vi "WS1050 16 DUT VSA-CV Sweep HD_Cycling_Ver1.2.vi"() -> ()   [LabVIEW 2012]
uses:
  WS_VCAP Driver 024/Source/WSVCAP Shell/Type Defs/WSVCAP SHL I2C DUT Mask Mode Enum.ctl
  <vilib>/Utility/file.llb/Read From Spreadsheet File (DBL).vi
panel:
  out "VISA resource name out":refnum<visa-resource-name>="GPIB0::3::INSTR"
  out "date string":string="5/19/2014"
  out "PS1 Out":refnum<visa-resource-name>
  out "Ke2000 Out":refnum<visa-resource-name>="GPIB0::9::INSTR"
  in  "Tab Control":enum32{"Inst Control", "Data Output", "Graphs"}(tab)
  in  "Bank to Stress":u16(ring) items=["All OFF", "All ON", "Bank_C1", "Bank_C2", "Bank_C3"]
  out "AD7747 Values":string[][](table)
  in  "Lot#":string="4NEMB"
  in  "Wafer#":string="20-EB"
  in  "File Name":string="HD_4NEMB_25_EB_65C_44V_100DC_BRD2_150916_1"
  in  "TMN DC\\CAP Data Log File Path":path=path "C:/WS1050 16 DUT Data"
  in  "SN":string[](array[string])=["1", "2", "3", "4", "5", "6", "7", "8", "9", "10", "11", "12", "13", "14", "15", "16"]
  in  "Test Program":string="WS1050 16 DUT VSA_CV Sweep HD_Cycling Ver1.2"
  out "Current Date":string="8/28/2014"
  out "Current Time":string="0950"
  in  "Start Date":string="4/24/2014"
  in  "Start Time":string="1542"
  in  "Comment":string="VSA CV Sweep"
  in  "OK Button":bool
  in  "Calibration":bool
  in  "Control Setting":bool
  in  "CP Setting":i32(ring) items=["CP OFF", "CP ON", "CP 35V", "CP 40V", "CP 44V", "CP 50V", "DVA OFF", "DVA ON", "Reg1 ON", "Reg1 OFF", "Reg2 ON", "Reg2 OFF", "Reg3 ON", "Reg3 OFF"]
  in  "VDD(V)":dbl=3.3 format="%.3g"
  in  "SPI Clock Rate (Hz)":dbl=1000000.0 caption="Meas Speed" format="%.1p Hz"
  out "AR  Measurent(Hz)":dbl
  in  "PS1 Source":refnum<visa-resource-name>="GPIB0::5::INSTR"
  in  "Ke2000":refnum<visa-resource-name>="GPIB0::9::INSTR"
  out "Simulate FPGA":bool
  out "Online":bool
  in  "Ke2400":refnum<visa-resource-name>="GPIB0::3::INSTR"
  in  "Initialize AD7747":bool
  in  "DUT Mask Mode":T1=enum."All"
  in  "RFFE Slave Address":u8=7 caption="Slave Address" format="0x%02x"
  out "Activity Log":string="05/19/2014 -- 12:24:35.853::WSVCAP::APP::Application Started\n05/19/2014 -- 12:24:37.606::WSVCAP::WSVCAP SHL::WR I2C-REG:0x0A;MASK:0xFFFFFFFFFFFF;C1 DATA:22:22:22:22:22:22:22:22:22:22:22:22:22:22:22:22;C2 DATA:22:22:22:22:22:22:22:22:22:22:22:22:22:22:22:22;C3 DATA:22:22:22:22:22:22:22:22:22:22:22:22:22:22:22:22\r\n05/19/2014 -- 12:24:37.773::WSVCAP::WSVCAP SHL::WR I2C-ST:0,0,4,1\r\n05/19/2014 -- 12:24:37.903::WSVCAP::WSVCAP SHL::RD I2C-BYTES:4;ADD:0x00;MASK:0xFFFFFFFFFFFF\r\n05/19/2014 -- 12:24:38.045::WSVCAP::WSVCAP SHL::RD I2C:C1 DATA:2:2:2:2:2:2:2:2:2:2:2:2:2:2:2:2|A7:A9:AA:82:82:7F:82:81:82:81:83:82:81:82:82:81|46:36:BB:88:44:A3:E9:2B:32:20:ED:25:BB:3D:68:B|2C:6A:EB:A7:22:56:FE:CC:36:82:D7:B0:3B:48:F9:CC;C2 DATA:2:2:2:2:2:2:2:2:2:2:2:2:2:2:2:2|94:94:94:80:80:80:80:80:81:7E:7E:81:80:7E:80:80|47:33:15:82:62:B:E8:1C:D7:C3:7D:41:7C:B7:4C:2A|C4:B4:AE:8:1E:D1:4E:37:11:C0:6F:63:42:9D:63:B5;C3 DATA:2:2:2:2:2:2:2:2:2:2:2:2:2:2:2:2|95:95:95:81:81:7E:81:80:84:7D:80:83:81:7E:7F:80|AB:C4:14:B5:7B:52:DF:C9:79:5D:5F:30:99:31:1E:F4|6E:5C:F7:A8:C3:EB:7B:EF:33:92:89:77:4D:67:75:DD;STATUS:0:0:4:0\r\n05/19/2014 -- 12:24:38.046::WSVCAP::WSVCAP SHL::WR I2C-REG:0x0A;MASK:0xFFFFFFFFFFFF;C1 DATA:22:22:22:22:22:22:22:22:22:22:22:22:22:22:22:22;C2 DATA:22:22:22:22:22:22:22:22:22:22:22:22:22:22:22:22;C3 DATA:22:22:22:22:22:22:22:22:22:22:22:22:22:22:22:22\r\n05/19/2014 -- 12:24:38.089::WSVCAP::WSVCAP SHL::WR I2C-ST:0,0,4,1\r\n05/19/2014 -- 12:24:38.219::WSVCAP::WSVCAP SHL::RD I2C-BYTES:4;ADD:0x00;MASK:0xFFFFFFFFFFFF\r\n05/19/2014 -- 12:24:38.362::WSVCAP::WSVCAP SHL::RD I2C:C1 DATA:2:2:2:2:2:2:2:2:2:2:2:2:2:2:2:2|A7:AB:AA:82:82:82:83:83:82:82:82:82:7F:82:82:81|4B:32:96:83:3E:61:43:17:25:62:AB:4D:A2:40:2E:5|3C:76:2B:B4:EE:E4:A9:1A:AA:A:26:C7:21:2E:87:5B;C2 DATA:2:2:2:2:2:2:2:2:2:2:2:2:2:2:2:2|94:94:94:80:80:80:80:80:80:7F:80:81:80:80:7F:80|4A:32:19:7D:19:6C:79:46:61:7F:4B:B8:A5:30:F3:14|B4:70:A:8C:9C:DC:43:FA:1E:A:C6:21:A:A9:13:F3;C3 DATA:2:2:2:2:2:2:2:2:2:2:2:2:2:2:2:2|95:97:94:81:80:81:82:81:80:7E:81:84:7F:81:80:80|B2:32:D0:A7:9E:4C:AB:D4:EE:D9:F0:82:B7:91:7:FF|C1:91:B6:3D:D8:E:1B:4F:9F:6A:F1:6C:E7:3F:7:BA;STATUS:0:0:4:0\r\n05/19/2014 -- 12:24:38.364::WSVCAP::WSVCAP SHL::WR I2C-REG:0x0A;MASK:0xFFFFFFFFFFFF;C1 DATA:22:22:22:22:22:22:22:22:22:22:22:22:22:22:22:22;C2 DATA:22:22:22:22:22:22:22:22:22:22:22:22:22:22:22:22;C3 DATA:22:22:22:22:22:22:22:22:22:22:22:22:22:22:22:22\r\n05/19/2014 -- 12:24:38.406::WSVCAP::WSVCAP SHL::WR I2C-ST:0,0,4,1\r\n05/19/2014 -- 12:24:38.536::WSVCAP::WSVCAP SHL::RD I2C-BYTES:4;ADD:0x00;MASK:0xFFFFFFFFFFFF\r\n05/19/2014 -- 12:24:38.678::WSVCAP::WSVCAP SHL::RD I2C:C1 DATA:2:2:2:2:2:2:2:2:2:2:2:2:2:2:2:2|A7:A9:AB:82:82:81:82:82:82:82:82:82:82:82:82:81|46:71:4C:87:43:3D:7F:FC:25:4F:8E:54:97:3E:60:8C|AA:F4:1F:B5:CE:43:1F:36:9:87:9C:78:86:5:B6:8E;C2 DATA:2:2:2:2:2:2:2:2:2:2:2:2:2:2:2:2|94:94:94:80:7F:7F:80:80:80:80:80:81:80:80:80:80|49:36:18:7D:6E:C5:E4:3C:81:2E:41:D3:75:71:E3:72|E8:D3:E6:D1:E0:48:AE:D4:54:D:E8:8E:B4:41:68:4;C3 DATA:2:2:2:2:2:2:2:2:2:2:2:2:2:2:2:2|95:95:95:81:7F:7F:81:81:81:81:81:84:81:81:82:81|B3:F5:90:AB:82:69:7B:93:D0:77:E8:D5:E8:8C:84:E8|B9:AC:EE:2B:B6:71:8F:4A:74:31:56:BB:8A:B7:A0:C8;STATUS:0:0:4:0\r\n05/19/2014 -- 12:24:38.681::WSVCAP::WSVCAP SHL::WR I2C-REG:0x0A;MASK:0xFFFFFFFFFFFF;C1 DATA:22:22:22:22:22:22:22:22:22:22:22:22:22:22:22:22;C2 DATA:22:22:22:22:22:22:22:22:22:22:22:22:22:22:22:22;C3 DATA:22:22:22:22:22:22:22:22:22:22:22:22:22:22:22:22\r\n05/19/2014 -- 12:24:38.723::WSVCAP::WSVCAP SHL::WR I2C-ST:0,0,4,1\r\n05/19/2014 -- 12:24:38.854::WSVCAP::WSVCAP SHL::RD I2C-BYTES:4;ADD:0x00;MASK:0xFFFFFFFFFFFF\r\n05/19/2014 -- 12:24:38.996::WSVCAP::WSVCAP SHL::RD I2C:C1 DATA:2:2:2:2:2:2:2:2:2:2:2:2:2:2:2:2|A7:A9:AA:82:82:7F:83:81:82:81:84:82:7F:82:7F:82|43:FB:E:7F:3C:AD:35:35:26:A2:6C:21:4B:3D:8:6|63:9A:E1:F3:95:32:91:42:90:3C:78:1F:5C:D7:5F:D8;C2 DATA:2:2:2:2:2:2:2:2:2:2:2:2:2:2:2:2|94:94:94:80:80:80:80:80:81:80:7E:81:80:7E:7F:80|48:36:18:7F:5E:3D:69:83:DE:AE:A1:9E:31:AE:BB:96|15:A0:44:17:13:FD:CC:C8:6D:B2:EF:A7:C:C7:3B:F;C3 DATA:2:2:2:2:2:2:2:2:2:2:2:2:2:2:2:2|95:96:94:81:81:7E:82:80:84:80:80:84:7F:7E:7D:82|AD:3B:6D:A9:7C:57:9D:F5:7A:96:23:5C:36:2D:ED:5A|CD:46:DB:3B:C7:BD:70:60:33:B8:B:F7:63:A:51:4D;STATUS:0:0:4:0\r\n05/19/2014 -- 12:24:38.998::WSVCAP::WSVCAP SHL::WR I2C-REG:0x0A;MASK:0xFFFFFFFFFFFF;C1 DATA:22:22:22:22:22:22:22:22:22:22:22:22:22:22:22:22;C2 DATA:22:22:22:22:22:22:22:22:22:22:22:22:22:22:22:22;C3 DATA:22:22:22:22:22:22:22:22:22:22:22:22:22:22:22:22\r\n05/19/2014 -- 12:24:39.040::WSVCAP::WSVCAP SHL::WR I2C-ST:0,0,4,1\r\n05/19/2014 -- 12:24:39.170::WSVCAP::WSVCAP SHL::RD I2C-BYTES:4;ADD:0x00;MASK:0xFFFFFFFFFFFF\r\n05/19/2014 -- 12:24:39.311::WSVCAP::WSVCAP SHL::RD I2C:C1 DATA:2:2:2:2:2:2:2:2:2:2:2:2:2:2:2:2|A7:AA:AB:82:82:81:82:81:82:81:82:82:82:82:7F:82|44:F1:90:87:45:44:C8:2C:2C:F1:FC:1B:94:3B:3C:75|4A:49:95:19:99:73:64:3:23:24:F3:A2:5E:7F:C4:B6;C2 DATA:2:2:2:2:2:2:2:2:2:2:2:2:2:2:2:2|94:94:94:80:80:80:80:7F:80:80:7E:80:80:7E:7F:80|4C:36:17:7D:A8:9F:DE:C7:53:6D:8A:F4:41:A5:C6:E0|90:2E:24:C:D9:22:E4:76:3B:40:1D:53:33:B1:3E:4D;C3 DATA:2:2:2:2:2:2:2:2:2:2:2:2:2:2:2:2|95:97:95:81:81:7F:81:80:80:81:7F:82:81:7E:7D:82|AE:2B:A7:AB:CC:CD:A4:38:FD:17:80:F2:92:2D:45:C4|76:E5:D:B9:AD:B5:BA:8D:28:32:9E:42:B7:20:4A:D9;STATUS:0:0:4:0\r\n05/19/2014 -- 12:24:39.313::WSVCAP::WSVCAP SHL::WR I2C-REG:0x0A;MASK:0xFFFFFFFFFFFF;C1 DATA:22:22:22:22:22:22:22:22:22:22:22:22:22:22:22:22;C2 DATA:22:22:22:22:22:22:22:22:22:22:22:22:22:22:22:22;C3 DATA:22:22:22:22:22:22:22:22:22:22:22:22:22:22:22:22\r\n05/19/2014 -- 12:24:39.355::WSVCAP::WSVCAP SHL::WR I2C-ST:0,0,4,1\r\n05/19/2014 -- 12:24:39.486::WSVCAP::WSVCAP SHL::RD I2C-BYTES:4;ADD:0x00;MASK:0xFFFFFFFFFFFF\r\n05/19/2014 -- 12:24:39.628::WSVCAP::WSVCAP SHL::RD I2C:C1 DATA:2:2:2:2:2:2:2:2:2:2:2:2:2:2:2:2|A7:A9:AA:82:82:82:83:82:82:82:82:82:7F:82:7F:82|47:18:E4:87:3E:E7:6:65:25:92:37:38:A8:3E:89:85|7C:A7:7:2B:A3:7A:EC:EF:89:ED:F4:D3:D8:BC:3A:F5;C2 DATA:2:2:2:2:2:2:2:2:2:2:2:2:2:2:2:2|94:94:94:80:7F:80:80:7F:81:80:7E:80:80:80:81:80|49:37:17:80:76:25:6A:F8:DF:55:97:4D:B8:5B:2B:B1|13:E3:9A:3E:1A:2D:4F:B6:DB:E9:61:FA:8B:D6:9:CC;C3 DATA:2:2:2:2:2:2:2:2:2:2:2:2:2:2:2:2|95:95:95:81:7F:80:82:81:84:80:7F:81:80:81:7F:82|AF:93:3B:AF:5B:11:82:E4:7E:C3:2D:72:9:96:D9:A|DB:96:F2:10:5F:64:9A:C6:98:12:27:7D:10:D3:20:D9;STATUS:0:0:4:0\r\n05/19/2014 -- 12:24:40.132::WSVCAP::WSVCAP SHL::CLOSE\r\n"
  in  "C1 Cap DAC":u8=128 caption="B Data In" format="0x%02x"
  in  "C2 Cap DAC":u8=128 caption="B Data In" format="0x%02x"
  in  "C3 Cap DAC":u8=128 caption="B Data In" format="0x%02x"
  out "IDD Brd(uA)":string
  in  "VSA_IDD(A)":dbl=0.1
  in  "Stress Voltage(V)":dbl=10.0
  in  "CP to HD/Cycle":i32(ring)=4 items=["CP HDC 35V", "CP HDC 40.25V", "CP HDC 27.5V", "CP HDC 30.5V", "CP HDC 44V", "CP HDC 50V"]
  in  "Reset PS":bool
  in  "CP Freq":u16(ring)=3 items=["000", "001", "010", "011", "100", "101", "110", "111"]
  out "STATUS":string="Idle...."
  in  "stop":bool
  out "C1 Min_T0":string[](array[string])
  out "CAP_Value(pF)":string[][](array[string])
  out "C3 Min_T0":string[](array[string])
  out "C2 Min_T0":string[](array[string])
  in  "Abort":bool
  out "error out 2":errorcluster
  in  "Set HD Time \nto Complete(Min)":u64=8100
  out "HD Time\nCompleted(Min)":u64
  out "Verify Test Condition":string[](array[string])
  out "CMin+VCAP":string[][](table)
  out "Previous Time":string="12:20:26 PM"
  out "Running Loops":i32=1
  out "Verify Drivers to Stress":string[](array[string])
  out "Delta CAP_T0(pF)":dbl[][](array[numeric])
  out "Delta CAP_Tc(pF)":dbl[][](array[numeric])
  in  "error in (no error)":errorcluster
  out "error out":errorcluster
  out "CP_IDD(uA)":string
  # "Company:  WiSpry Inc 20 Fairbanks \nSte 198 Irvine CA 92618\n\nAuthor:  Andy V Tran\nCreated:  01/05/2016\nLabVIEW 2012 Pro\nTP:  WS1050 16 DUT VSA_CV Sweep HD_Cycling Ver1.2\nFPGA Version: WS_VCAP Driver 024"
  # "Note:  Ver1.0 is a original version.\n\n1.  Two look up tables, \n      a.  1st is for Stress\n      b.  2nd is for Voltage sweep\n\nVer1.1\n\n1.  No Voltage to CAP Head for initial read point\n\nVer1.2\n\n1.  Add CP Freq\n\nSet up and Test Sequences:\n\n1.  Calibration with Empty Sockets\n2.  Load Parts\n3.  Set condition to stress (CP Voltage, Drivers to Stress, CP to stress...)\n4.  Set Date/Time to start stressing\n5.  Set TTF to stop stressing (default = 135 hrs)"
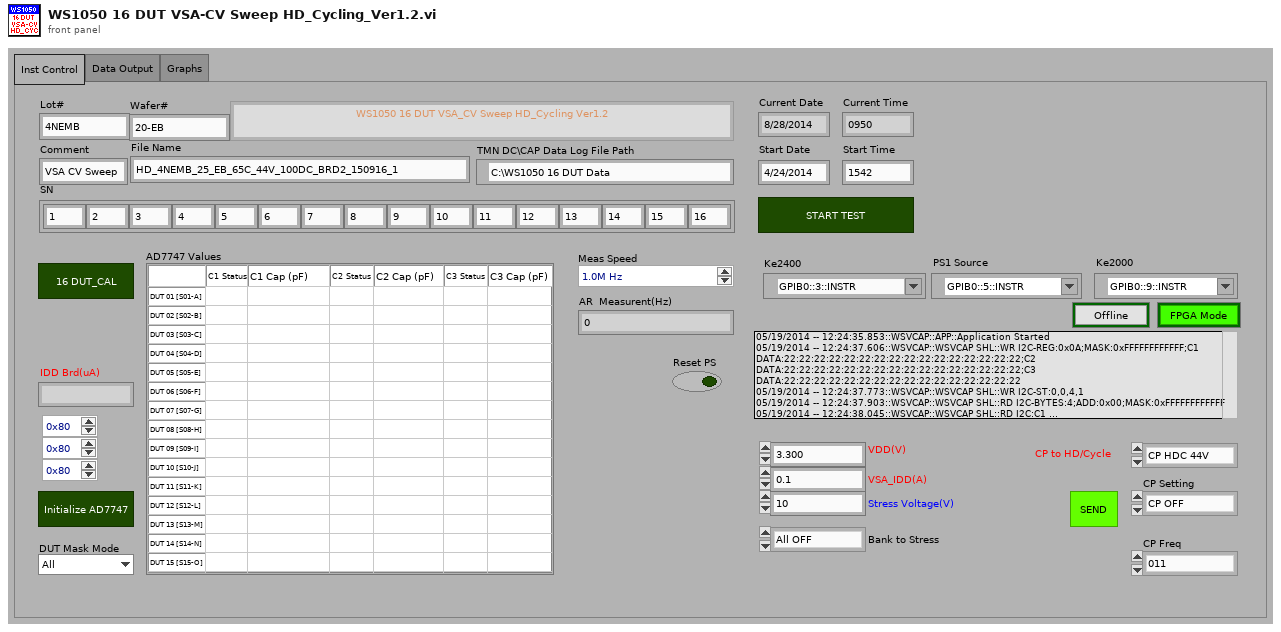
[diagram p1: front panel]
types:
  T1 = typedef "WSVCAP SHL I2C DUT Mask Mode Enum.ctl" = enum16{"Custom", "C1", "C2", "C3", "All"}
  T2 = typedef "WSVCAP SHL Core System Cluster.ctl" = cluster{"Settings":T3, "FPGA Resource":tag, "Online":bool, "I2C Wait Ticks":u32, "SPI Wait Ticks":u32, "RFFE Wait Ticks":u32}
  T3 = typedef "WSVCAP SHL I2C Settings Cluster.ctl" = cluster{"FPGA Resource Name":string, "I2C Slave Address":u8, "I2C Clock Rate (Hz)":dbl, "SPI Clock Rate (Hz)":dbl, "RFFE Slave Address":u8, "RFFE Clock Rate (Hz)":dbl, "Simulate FPGA":bool, "C1 Cap DAC Default":u8, "C2 Cap DAC Default":u8, "C3 Cap DAC Default":u8}
  T4 = enum16{"Idle...", "Voltage 1", "Voltage 2", "Voltage 3"}[]
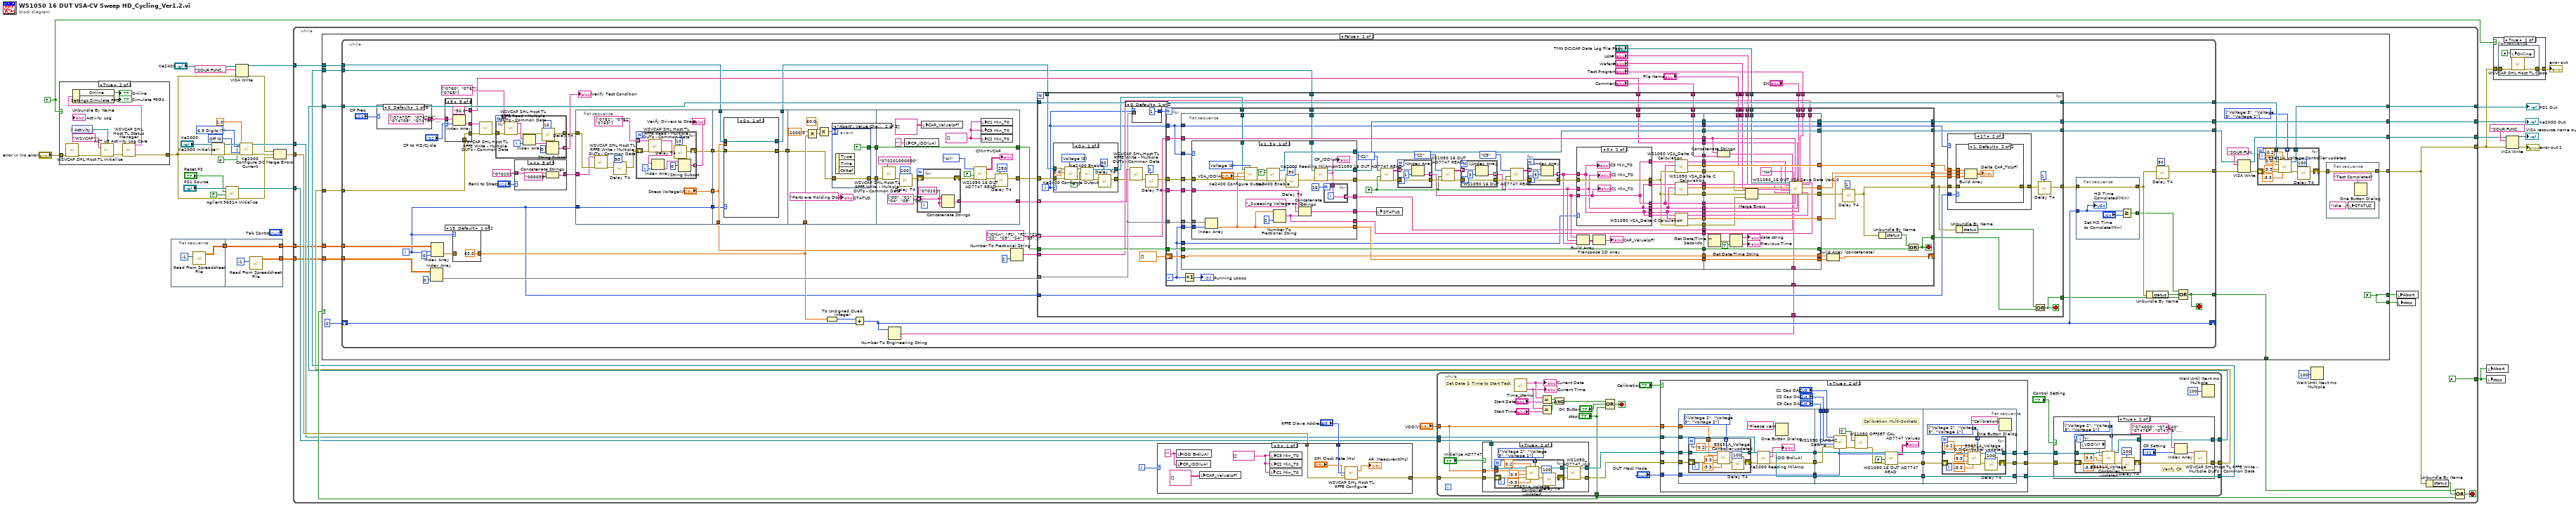
[diagram p0: block diagram]
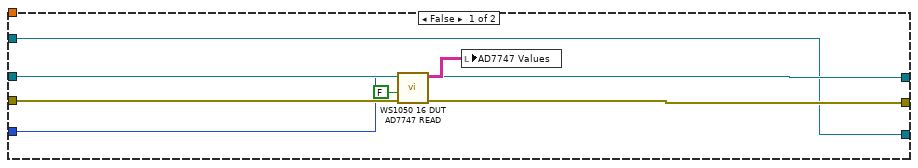
[diagram p7: hidden frame]
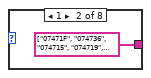
[diagram p8: hidden frame]
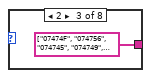
[diagram p9: hidden frame]
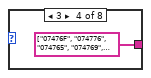
[diagram p10: hidden frame]
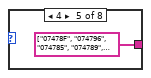
[diagram p11: hidden frame]
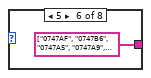
[diagram p12: hidden frame]
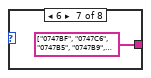
[diagram p13: hidden frame]
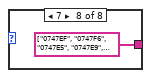
[diagram p14: hidden frame]
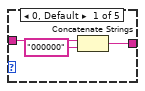
[diagram p15: hidden frame]
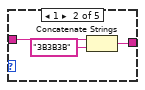
[diagram p16: hidden frame]
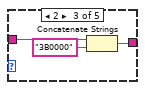
[diagram p17: hidden frame]
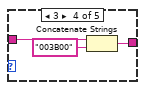
[diagram p18: hidden frame]
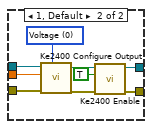
[diagram p20: hidden frame]
diagram:
  w21 = TRUE
  w27 = u16 0 items=["Off", "Moving Filter", "Repeating Filter"] ("Digital Filter (0: Off)")
  w28 = u16 7 items=["3.5 Digits"=4, "4.5 Digits"=5, "5.5 Digits"=6, "6.5 Digits"=7] ("Resolution (7: 6.5 digits)")
  n1 = case shown="True" w21 {
    tunnel: "error in (no error)" -> [w35 w36]
    tunnel: [w35 w43] -> w10
    frame False {
    }
    frame True {
      n2 = call "WSVCAP SHL Host TL Initialize.vi"("error in"=w36) -> ("error out"=w37:errorcluster)  [unwired: 13 in, 1 out]
      n3 = control-ref of="Activity Log"() -> (w39:refnum<vi>)
      n4 = call "ACT LG Activity Log Core.vi"("Display Ref"=w39, "Source"="WSVCAP", "Error In (no error)"=w37) -> ("Error Out"=w38:errorcluster)  [unwired: 11 in, 1 out]
      n5 = call "WSVCAP SHL Host TL Status Manager.vi"("error in"=w38) -> ("System Out"=w44:T2, "error out"=w43:errorcluster)  [unwired: 13 in]
      n6 = Unbundle By Name(w44) -> ("Online"=→"Online":bool, "Settings.Simulate FPGA"=→"Simulate FPGA":bool)
    }
  }
  n7 = flat-sequence {
    tunnel: [w46] -> w5
    tunnel: w5 -> [w49]
    tunnel: [w49] -> w4
    tunnel: [w48] -> w3
    frame #0 {
      n8 = call-poly <vilib>:"Read From Spreadsheet File.vi"("number of rows (all:-1)"=-1) -> ("all rows"=w46:dbl[][])  [unwired: 6 in, 4 out]
    }
    frame #1 {
      n9 = call-poly <vilib>:"Read From Spreadsheet File.vi"("number of rows (all:-1)"=-1) -> ("all rows"=w48:dbl[][])  [unwired: 6 in, 4 out]
    }
  }
  n10 = call "Ke2000 Initialize.vi"("error in (no error)"=w10, "VISA resource name"="Ke2000") -> ("error out"=w29:errorcluster, "VISA resource name out"=w30:refnum<visa-resource-name>)  [unwired: 8 in]
  n11 = call "Agilent 3631A Initialize.vi"("error in (no error)"=w10, "Default"=FALSE ("Reset? (T: Yes)"), "Reset"="Reset PS", "VISA resource name"="PS1 Source") -> ("error out"=w9:errorcluster, "VISA resource name out"=w33:refnum<visa-resource-name>)  [unwired: 6 in]
  n12 = VISA Write(VISA resource name="Ke2400", write buffer="SOUR:FUNC VOLT;VOLT:MODE FIX;RANG 100;LEV 0.0;:SENS:FUNC \"CURR\";CURR:PROT 60E-3;RANG 100E-3;:OUTP ON", error in (no error)=w10) -> (VISA resource name out=w18:refnum<visa-resource-name>, error out=w13:errorcluster)  [unwired: 1 out]
  n13 = call "Ke2000 Configure DC Current.vi"("Resolution (7: 6.5 digits)"=w28, "Digital Filter (0: Off)"=w27, "Auto Range? (T: Auto)"=FALSE, "error in"=w29, "Custom Range (0 A)"=1.0, "VISA resource name"=w30) -> ("error out"=w11:errorcluster, "VISA resource name out"=w25:refnum<visa-resource-name>)  [unwired: 4 in]
  n14 = Merge Errors(w13, w11, w9) -> (w19:errorcluster)
  n15 = while {
    tunnel: w19 -> [w68]
    tunnel: [w57] -> w15
    tunnel: w33 -> [w61]
    tunnel: w25 -> [w62]
    tunnel: [w71] -> w24
    tunnel: [w70] -> w23
    tunnel: w18 -> [w67]
    tunnel: [w66] -> w16
    tunnel: [FALSE] -> w8
    tunnel: w4 -> [w53]
    tunnel: w3 -> [w52]
    i -> [w69]
    stop <- w72 stop-if-true
    n16 = case shown="0" w69 {
      tunnel: w68 -> [w82 w83]
      tunnel: [w81 w83] -> w64
      tunnel: "RFFE Slave Address" -> [w79 _]
      frame 0 {
        w77 = string[] []
        w75 = "" ("uA")
        n17 = local write "IDD Brd(uA)"(w75) -> ()
        n18 = local write "CP_IDD(uA)"(w75) -> ()
        n19 = local write "CAP_Value(pF)"(string[][] []) -> ()
        n20 = local write "C1 Min_T0"(w77) -> ()
        n21 = local write "C3 Min_T0"(w77) -> ()
        n22 = local write "C2 Min_T0"(w77) -> ()
        n23 = call "WSVCAP SHL Host TL RFFE Configure.vi"("RFFE Slave Address"=w79, "Clock Rate (Hz)"="SPI Clock Rate (Hz)", "error in"=w82) -> ("Actual Rate (Hz)"=→"AR  Measurent(Hz)":dbl, "error out"=w81:errorcluster)  [unwired: 11 in]
      }
      frame 1, Default {
      }
    }
    n24 = while {
      tunnel: ["stop"] -> w65
      tunnel: w64 -> [w95]
      tunnel: [w87] -> w58
      tunnel: w61 -> [w93]
      tunnel: w62 -> [w89]
      tunnel: [w90] -> w60
      tunnel: [w88] -> w59
      tunnel: "VDD(V)" -> [w85]
      stop <- w102 stop-if-true
      # "Set Date & Time to Start Test"
      n25 = case shown="True" "Initialize AD7747" {
        tunnel: w95 -> [w111 w117]
        tunnel: [w111 w113] -> w94
        tunnel: w93 -> [w110 w115]
        tunnel: [w110 w114] -> w92
        tunnel: w85 -> [_ w112]
        frame False {
        }
        frame True {
          w118 = T4 [enum."Voltage 2", enum."Voltage 3", enum."Voltage 1"] items=["Idle...", "Voltage 1", "Voltage 2", "Voltage 3"]
          n26 = for {
            tunnel: w115 -> [w128]
            tunnel: w118 -> [w126] mode=indexing
            tunnel: [w125] -> w114
            shift-right: [w122] -> w116
            shift-left: w117 -> [w129]
            tunnel: w112 -> [w120]
            n27 = call "E3631A_Voltage Controller updated.vi"("VISA resource name"=w128, "I_VDD(A)"=0.2, "Channel Controller"=w126, "Voltage 1"=w120, "Voltage 2"=3.3, "error in (no error)"=w129, "Voltage 3"=-3.3) -> ("VISA resource name out"=w125:refnum<visa-resource-name>, "error out"=w121:errorcluster)  [unwired: 7 in]
            n28 = call "Delay T4.vi"("milliseconds to wait"=u32 100, "error in (no error)"=w121) -> ("error out"=w122:errorcluster)  [unwired: 9 in]
          }
          n29 = call "WS1050_AD7747_Init.vi"("error in"=w116) -> ("error out"=w113:errorcluster)  [unwired: 10 in]
        }
      }
      n30 = call "Time_stamp.vi"() -> ("date/time string"=w107:string, "date string"=w109:string)  [unwired: 2 in]
      "Current Date" <- w109
      "Current Time" <- w107
      n31 = Equal?(x=w109, y="Start Date") -> (x = y?=w105:bool)
      n32 = Equal?(x=w107, y="Start Time") -> (x = y?=w104:bool)
      n33 = And(x=w105, y=w104) -> (x .and. y?=w101:bool)
      n34 = Compound Arithmetic op=OR(w101, "OK Button", "stop") -> (w102:bool)
      n35 = case shown="True" "Calibration" {
        tunnel: w94 -> [w156 w175]
        tunnel: [w155 w172] -> w86
        tunnel: w92 -> [w154 w171]
        tunnel: "DUT Mask Mode" -> [w153 w167]
        tunnel: [w154 w166] -> w91
        tunnel: w89 -> [w152 w162]
        tunnel: [w152 w159] -> w88
        tunnel: w85 -> [_ w158]
        frame False {
          n36 = call "WS1050 16 DUT AD7747 READ.vi"("error in"=w156, "Log (T)"=FALSE, "DUT Mask Mode (All)"=w153) -> ("error out"=w155:errorcluster, "AD7747 Values"=w157:string[][])  [unwired: 7 in]
          n37 = local write "AD7747 Values"(w157) -> ()
        }
        frame True {
          n38 = flat-sequence {
            tunnel: w175 -> [w185]
            tunnel: [w180] -> w174
            tunnel: w171 -> [w184]
            tunnel: [w183] -> w170
            tunnel: w167 -> [w182]
            tunnel: [w182] -> w168
            tunnel: w162 -> [w178]
            tunnel: [w177] -> w161
            tunnel: w158 -> [w176]
            tunnel: w174 -> [w211]
            tunnel: [w210] -> w173
            tunnel: w170 -> [w209]
            tunnel: [w209] -> w169
            tunnel: w168 -> [w208]
            tunnel: "C1 Cap DAC" -> [w204]
            tunnel: "C2 Cap DAC" -> [w203]
            tunnel: "C3 Cap DAC" -> [w202]
            tunnel: w161 -> [w201]
            tunnel: [w201] -> w160
            tunnel: w173 -> [w214]
            tunnel: [w217] -> w172
            tunnel: w169 -> [w216]
            tunnel: [w213] -> w166
            tunnel: w160 -> [w212]
            tunnel: [w212] -> w159
            frame #0 {
              w186 = T4 [enum."Voltage 2", enum."Voltage 3", enum."Voltage 2"] items=["Idle...", "Voltage 1", "Voltage 2", "Voltage 3"]
              n39 = for {
                tunnel: w184 -> [w197]
                tunnel: w186 -> [w194] mode=indexing
                tunnel: [w193] -> w183
                shift-right: [w191] -> w179
                shift-left: w185 -> [w198]
                tunnel: w176 -> [w188]
                n40 = call "E3631A_Voltage Controller updated.vi"("VISA resource name"=w197, "I_VDD(A)"=0.2, "Channel Controller"=w194, "Voltage 1"=w188, "Voltage 2"=3.3, "error in (no error)"=w198, "Voltage 3"=-3.3) -> ("VISA resource name out"=w193:refnum<visa-resource-name>, "error out"=w190:errorcluster)  [unwired: 7 in]
                n41 = call "Delay T4.vi"("milliseconds to wait"=u32 100, "error in (no error)"=w190) -> ("error out"=w191:errorcluster)  [unwired: 9 in]
              }
              n42 = call "Ke2000 Reading MilAmp.vi"("error in (no error)"=w179, "VISA resource name"=w178) -> ("error out"=w180:errorcluster, "uA"=→"IDD Brd(uA)":string, "VISA resource name out"=w177:refnum<visa-resource-name>)  [unwired: 7 in]
              n43 = One Button Dialog(message="Please verify all sockets should be empty...") -> ()  [unwired: 1 in, 1 out]
            }
            frame #1 {
              # "Calibration Multi-Sockets"
              n44 = call "WS1050 CAPDAC Setting.vi"("DUT Mask Mode (All)"=w208, "error in"=w211, "C3 Cap DAC"=w202, "C2 Cap DAC"=w203, "C1 Cap DAC"=w204) -> ("error out"=w206:errorcluster)  [unwired: 5 in, 1 out]
              n45 = call "WS1050 OFFSET CAL.vi"("error in"=w206, "OFFSET CAL"=TRUE ("Read?")) -> ("error out"=w205:errorcluster)  [unwired: 8 in, 1 out]
              n46 = call "WS1050 16 DUT AD7747 READ.vi"("error in"=w205, "Log (T)"=FALSE, "DUT Mask Mode (All)"=w208) -> ("error out"=w210:errorcluster, "AD7747 Values"=→"AD7747 Values":string[][])  [unwired: 7 in]
            }
            frame #2 {
              w215 = T4 [enum."Voltage 2", enum."Voltage 3", enum."Voltage 1"] items=["Idle...", "Voltage 1", "Voltage 2", "Voltage 3"]
              n47 = for {
                tunnel: w216 -> [w229]
                tunnel: w215 -> [w225] mode=indexing
                tunnel: [w224] -> w213
                shift-right: [w220] -> w217
                shift-left: w214 -> [w226]
                n48 = call "E3631A_Voltage Controller updated.vi"("VISA resource name"=w229, "I_VDD(A)"=0.2, "Channel Controller"=w225, "Voltage 1"=0.0, "Voltage 2"=3.3, "error in (no error)"=w226, "Voltage 3"=-3.3) -> ("VISA resource name out"=w224:refnum<visa-resource-name>, "error out"=w219:errorcluster)  [unwired: 7 in]
                n49 = call "Delay T4.vi"("milliseconds to wait"=u32 100, "error in (no error)"=w219) -> ("error out"=w220:errorcluster)  [unwired: 9 in]
              }
              n50 = One Button Dialog(message="Calibration Completed....") -> ()  [unwired: 1 in, 1 out]
            }
          }
        }
      }
      n51 = case shown="True" "Control Setting" {
        tunnel: [w130 w133] -> w87
        tunnel: w91 -> [w131 w136]
        tunnel: [w131 w134] -> w90
        tunnel: w86 -> [w130 w132]
        frame False {
        }
        frame True {
          w137 = T4 [enum."Voltage 2", enum."Voltage 3", enum."Voltage 1"] items=["Idle...", "Voltage 1", "Voltage 2", "Voltage 3"]
          # "Verify CP"
          n52 = for {
            tunnel: w136 -> [w149]
            tunnel: w137 -> [w146] mode=indexing
            shift-right: [w143] -> w135
            shift-left: w132 -> [w150]
            tunnel: [w141] -> w134
            n53 = local read "VDD(V)"() -> (w145:dbl)
            n54 = call "E3631A_Voltage Controller updated.vi"("VISA resource name"=w149, "Channel Controller"=w146, "Voltage 1"=w145, "Voltage 2"=3.3, "error in (no error)"=w150, "Voltage 3"=-3.3) -> ("VISA resource name out"=w141:refnum<visa-resource-name>, "error out"=w144:errorcluster)  [unwired: 8 in]
            n55 = call "Delay T4.vi"("milliseconds to wait"=u32 100, "error in (no error)"=w144) -> ("error out"=w143:errorcluster)  [unwired: 9 in]
          }
          n56 = Index Array(array=string[] ["074000", "074040", "07476F", "074776", "07477B", "07477C", "074820", "074800", "07413B", "074100", "07423B", "074200", "07433B", "074300"], index="CP Setting") -> (element=w138:string)
          n57 = call "WSVCAP SHL Host TL RFFE Write - Multiple DUTs - Common Data.vi"("Data Out"=w138, "error in"=w135) -> ("error out"=w133:errorcluster)  [unwired: 13 in]
        }
      }
      n58 = Wait Until Next ms Multiple(millisecond multiple=u32 100) -> ()  [unwired: 1 out]
    }
    n59 = case shown="False" w65 {
      tunnel: w58 -> [w246 w757]
      tunnel: [w230 w757] -> w57
      tunnel: w60 -> [w244 w755]
      tunnel: w59 -> [w247 w756]
      tunnel: [w243 w756] -> w71
      tunnel: [w234 w755] -> w70
      tunnel: w67 -> [w249 w754]
      tunnel: [w245 w754] -> w66
      tunnel: [w242 w753] -> w55
      tunnel: [w242 w753] -> w54
      tunnel: w53 -> [w240 _]
      tunnel: w52 -> [w238 _]
      tunnel: [w233 w753] -> w50
      frame False {
        w237 = T4 [enum."Voltage 3", enum."Voltage 3", enum."Voltage 1"] items=["Idle...", "Voltage 1", "Voltage 2", "Voltage 3"]
        w242 = FALSE
        n60 = while {
          tunnel: w249 -> [w278]
          tunnel: w247 -> [w274]
          tunnel: w246 -> [w269]
          tunnel: w244 -> [w316]
          tunnel: [w315] -> w243
          tunnel: [w314] -> w235
          tunnel: [w313] -> w241
          tunnel: [w312] -> w232
          tunnel: w240 -> [w304]
          shift-right: [w295] -> _
          shift-left: u64 0 ("disabled index (col)") -> [w301]
          tunnel: w238 -> [w293]
          tunnel: [w268] -> w233
          i -> [w266]
          stop <- w268 stop-if-true
          n61 = case shown="0, Default" "CP Freq" {
            tunnel: [string[] ["07470F", "074716", "074705", "074709", "07471B", "07471C"] string[] ["07471F", "074736", "074715", "074719", "07473B", "07473C"] string[] ["07474F", "074756", "074745", "074749", "07475B", "07475C"] string[] ["07476F", "074776", "074765", "074769", "07477B", "07477C"] string[] ["07478F", "074796", "074785", "074789", "07479B", "07479C"] string[] ["0747AF", "0747B6", "0747A5", "0747A9", "0747BB", "0747BC"] string[] ["0747BF", "0747C6", "0747B5", "0747B9", "0747CB", "0747CC"] string[] ["0747EF", "0747F6", "0747E5", "0747E9", "0747FB", "0747FC"]] -> w262
            frame 0, Default {
            }
            frame 1 {
            }
            frame 2 {
            }
            frame 3 {
            }
            frame 4 {
            }
            frame 5 {
            }
            frame 6 {
            }
            frame 7 {
            }
          }
          n62 = Index Array(array=w293, index (col)=0 ("disabled index (col)")) -> (element=w292:dbl[])  [unwired: 1 in]
          n63 = Index Array(array=w304, index (row)=w266, index (col)=0 ("disabled index (col)")) -> (element=w282:dbl)
          n64 = case shown="5" "CP to HD/Cycle" {
            selector: "CP to HD/Cycle" -> [w436 w441 w446 w451 w456 w460]
            tunnel: w262 -> [w437 w442 w447 w452 w457 w462]
            tunnel: [w435 w440 w445 w450 w455 w461] -> w309
            tunnel: ["35.0" ("Data Out") "27.5" ("Data Out") "30.5" ("Data Out") "44.0" ("Data Out") "50.0" ("Data Out") "40.25" ("Data Out")] -> w288
            tunnel: [w433 w438 w443 w448 w453 w458] -> w308
            tunnel: w269 -> [w433 w438 w443 w448 w453 w458]
            frame 0, Default {
              n65 = Index Array(array=w437, index=w436) -> (element=w435:string)
            }
            frame 2 {
              n66 = Index Array(array=w442, index=w441) -> (element=w440:string)
            }
            frame 3 {
              n67 = Index Array(array=w447, index=w446) -> (element=w445:string)
            }
            frame 4 {
              n68 = Index Array(array=w452, index=w451) -> (element=w450:string)
            }
            frame 5 {
              n69 = Index Array(array=w457, index=w456) -> (element=w455:string)
            }
            frame 1 {
              n70 = Index Array(array=w462, index=w460) -> (element=w461:string)
            }
          }
          n71 = case shown="15, Default" w266 {
            tunnel: w282 -> [_ w346]
            tunnel: [60.0 w346] -> w281
            frame 15, Default {
            }
            frame 0..14 {
            }
          }
          n72 = call "WSVCAP SHL Host TL RFFE Write - Multiple DUTs - Common Data.vi"("Data Out"=w309, "error in"=w308) -> ("error out"=w306:errorcluster)  [unwired: 13 in]
          n73 = for {
            tunnel: string[] ["0760", "0767", "0768"] -> [w432] mode=indexing
            tunnel: [w428] -> w305 mode=indexing
            tunnel: w306 -> [w426]
            tunnel: [w424] -> w299
            i -> [w431]
            n74 = call "WSVCAP SHL Host TL RFFE Read - Multiple DUTs - Common Data.vi"("Data Out"=w432, "error in"=w426) -> ("RFFE Data In"=w430:string[], "error out"=w423:errorcluster)  [unwired: 12 in]
            n75 = Index Array(array=w430, index=w431) -> (element=w427:string)
            n76 = call "Delay T4.vi"("milliseconds to wait"=u32 10, "error in (no error)"=w423) -> ("error out"=w424:errorcluster)  [unwired: 9 in]
            n77 = String Subset(string=w427, offset (0)=0) -> (substring=w428:string)  [unwired: 1 in]
          }
          "Verify Test Condition" <- w305
          n78 = case shown="4" "Bank to Stress" {
            tunnel: "070201" -> [w332 w334 w337 w340 w343]
            tunnel: [w330 w333 w336 w339 w342] -> w263
            frame 0, Default {
              n79 = Concatenate Strings(w332, "000000" ("string")) -> (w330:string)
            }
            frame 1 {
              n80 = Concatenate Strings(w334, "3B3B3B" ("string")) -> (w333:string)
            }
            frame 2 {
              n81 = Concatenate Strings(w337, "3B0000" ("string")) -> (w336:string)
            }
            frame 3 {
              n82 = Concatenate Strings(w340, "003B00" ("string")) -> (w339:string)
            }
            frame 4 {
              n83 = Concatenate Strings(w343, "00003B" ("string")) -> (w342:string)
            }
          }
          n84 = flat-sequence {
            tunnel: [w354] -> w280
            tunnel: w299 -> [w360]
            tunnel: ["Stress Voltage(V)"] -> w277
            tunnel: w266 -> [w352]
            tunnel: [w352] -> w267
            tunnel: w263 -> [w351]
            tunnel: w280 -> [w375]
            tunnel: [w376] -> w279
            tunnel: w278 -> [w374]
            tunnel: [w373] -> w276
            tunnel: w277 -> [w372]
            tunnel: [w372] -> w272
            tunnel: w267 -> [w371]
            tunnel: w279 -> [w390]
            tunnel: w281 -> [w392]
            tunnel: [w391] -> w287
            tunnel: [w389] -> w286
            tunnel: [w405] -> w285
            tunnel: [w418] -> w291
            tunnel: w287 -> [w418]
            tunnel: w286 -> [w414]
            tunnel: [w416] -> w275
            frame #0 {
              n85 = call "WSVCAP SHL Host TL RFFE Write - Multiple DUTs - Common Data.vi"("Data Out"=w351, "error in"=w360) -> ("error out"=w359:errorcluster)  [unwired: 13 in]
              n86 = call "Delay T4.vi"("milliseconds to wait"=u32 50, "error in (no error)"=w359) -> ("error out"=w356:errorcluster)  [unwired: 9 in]
              n87 = for {
                tunnel: string[] ["0761", "0762", "0763"] -> [w370] mode=indexing
                tunnel: [w366] -> w355 mode=indexing
                shift-right: [w363] -> w354
                shift-left: w356 -> [w369]
                i -> [w368]
                n88 = call "WSVCAP SHL Host TL RFFE Read - Multiple DUTs - Common Data.vi"("Data Out"=w370, "error in"=w369) -> ("RFFE Data In"=w365:string[], "error out"=w362:errorcluster)  [unwired: 12 in]
                n89 = Index Array(array=w365, index=w368) -> (element=w364:string)
                n90 = call "Delay T4.vi"("milliseconds to wait"=u32 10, "error in (no error)"=w362) -> ("error out"=w363:errorcluster)  [unwired: 9 in]
                n91 = String Subset(string=w364, offset (0)=0) -> (substring=w366:string)  [unwired: 1 in]
              }
              "Verify Drivers to Stress" <- w355
            }
            frame #1 {
              n92 = case shown="0" w371 {
                tunnel: [w377 w384] -> w376
                tunnel: w375 -> [w377 w383]
                tunnel: w374 -> [w378 w382]
                tunnel: [w378 w381] -> w373
                tunnel: w372 -> [_ w379]
                frame 0 {
                }
                frame 1, Default {
                  w380 = u16 0 items=["Voltage", "Current"] ("Source Mode  (0: Voltage)")
                  n93 = call "Ke2400 Configure Output.vi"("Source Mode  (0: Voltage)"=w380, "error in (no error)"=w383, "Output Level (0)"=w379, "VISA resource name"=w382) -> ("error out"=w387:errorcluster, "VISA resource name out"=w385:refnum<visa-resource-name>)  [unwired: 6 in]
                  n94 = call "Ke2400 Enable.vi"("error in (no error)"=w387, "ON/OFF"=TRUE ("Enable Output (T: Enable)"), "VISA resource name"=w385) -> ("error out"=w384:errorcluster, "VISA resource name out"=w381:refnum<visa-resource-name>)  [unwired: 7 in]
                }
              }
            }
            frame #2 {
              n95 = Multiply(x=1000.0, y=w392) -> (x*y=w395:dbl)
              n96 = Multiply(x=60.0, y=w395) -> (x*y=w396:dbl)
              n97 = event shown="[1] \"Abort\": Value Change" {
                selector: _ -> [_ _]
                dyn-events: _ -> [_ _]
                timeout: w396 -> [_ _]
                tunnel: ["Abort" TRUE ("Abort")] -> w391
                tunnel: w390 -> [w397 w399]
                tunnel: [w397 w399] -> w389
                event Timeout {
                  n98 = event-data() -> ()  [unwired: 1 in, 2 out]
                }
                event "Abort": Value Change {
                  n99 = event-data() -> ()  [unwired: 1 in, 3 out]
                }
              }
              "STATUS" <- "Parts are Holding Down...." ("STATUS")
            }
            frame #3 {
              w412 = string[] [] ("CP Current(uA)")
              n100 = call "WSVCAP SHL Host TL RFFE Write - Multiple DUTs - Common Data.vi"("Data Out"="070201000000", "error in"=w414) -> ("error out"=w408:errorcluster)  [unwired: 13 in]
              n101 = call "Delay T4.vi"("milliseconds to wait"=u32 100, "error in (no error)"=w408) -> ("error out"=w409:errorcluster)  [unwired: 9 in]
              n102 = local write "CP_IDD(uA)"("" ("CP_IDD(uA)")) -> ()
              n103 = for {
                tunnel: string[] ["00", "01", "02", "04", "08", "0C", "10", "14", "18", "1C", "20", "24", "28", "2C", "30", "34", "38", "3B", "00"] -> [w421] mode=indexing
                tunnel: [w420] -> w416 mode=indexing
                shift-right: [w419] -> w413
                shift-left: w409 -> [w419]
                n104 = Concatenate Strings("070201" ("string"), w421, w421, w421) -> (w420:string)
              }
              n105 = local write "CAP_Value(pF)"(string[][] [] ("VSA_Value(pF)")) -> ()
              n106 = call "WS1050 16 DUT AD7747 READ.vi"("error in"=w413, "Log (T)"=FALSE, "DUT Mask Mode (All)"=WSVCAP_SHL_I2C_DUT_Mask_Mode_Enum."All") -> ("error out"=w404:errorcluster, "AD7747 Values"=→"CMin+VCAP":string[][])  [unwired: 7 in]
              n107 = local write "C1 Min_T0"(w412) -> ()
              n108 = local write "C3 Min_T0"(w412) -> ()
              n109 = local write "C2 Min_T0"(w412) -> ()
              n110 = call "Delay T4.vi"("milliseconds to wait"=u32 250, "error in (no error)"=w404) -> ("error out"=w405:errorcluster)  [unwired: 9 in]
            }
          }
          n111 = To Unsigned Quad Integer(1:w281) -> (0:w302:u64)
          n112 = Add(x=w302, y=w301) -> (x+y=w295:u64)
          n113 = Number To Engineering String(4:w295) -> (0:w289:string)  [unwired: 3 in]
          n114 = Number To Fractional String(number=w272, precision (6)=i16 2) -> (F-format string=w271:string)  [unwired: 2 in]
          n115 = for {
            tunnel: w285 -> [w478]
            tunnel: [w502] -> w313
            tunnel: [w485] -> w298
            tunnel: "Comment" -> [w500]
            tunnel: "Lot#" -> [w499]
            tunnel: "Wafer#" -> [w498]
            tunnel: "SN" -> [w497]
            tunnel: "File Name" -> [w496]
            tunnel: [w495] -> w314
            tunnel: w316 -> [w495]
            tunnel: [w494] -> w315
            tunnel: w292 -> [w491]
            tunnel: w291 -> [w490]
            tunnel: [w487] -> w290
            tunnel: w289 -> [w470]
            tunnel: w288 -> [w486]
            tunnel: "TMN DC\\CAP Data Log File Path" -> [w483]
            tunnel: "Test Program" -> [w482]
            tunnel: w276 -> [w476]
            tunnel: w275 -> [w480] mode=indexing
            tunnel: w274 -> [w475]
            tunnel: string[] ["CMin", "F1", "F2", "S1", "S2", "S3", "S4", "S5", "S6", "S7", "S8", "S9", "S10", "S11", "S12", "S13", "S14", "S14F12", "All OFF"] -> [w473] mode=indexing
            tunnel: w271 -> [w474]
            tunnel: w266 -> [w464]
            i -> [w471]
            stop <- w487 stop-if-true
            n116 = case shown="0" w471 {
              tunnel: [w525 w535] -> w479
              tunnel: w478 -> [w532 w535]
              tunnel: [w531 w534] -> w477
              tunnel: w476 -> [w530 w534]
              frame 0 {
                w528 = u16 0 items=["Voltage", "Current"] ("Source Mode  (0: Voltage)")
                n117 = call "Ke2400 Configure Output.vi"("Source Mode  (0: Voltage)"=w528, "error in (no error)"=w532, "Output Level (0)"=0.0, "VISA resource name"=w530) -> ("error out"=w533:errorcluster, "VISA resource name out"=w526:refnum<visa-resource-name>)  [unwired: 6 in]
                n118 = call "Ke2400 Enable.vi"("error in (no error)"=w533, "ON/OFF"=TRUE ("Enable Output (T: Enable)"), "VISA resource name"=w526) -> ("error out"=w524:errorcluster, "VISA resource name out"=w531:refnum<visa-resource-name>)  [unwired: 7 in]
                n119 = call "Delay T4.vi"("milliseconds to wait"=u32 50, "error in (no error)"=w524) -> ("error out"=w525:errorcluster)  [unwired: 9 in]
              }
              frame 1, Default {
              }
            }
            n120 = call "WSVCAP SHL Host TL RFFE Write - Multiple DUTs - Common Data.vi"("Data Out"=w480, "error in"=w479) -> ("error out"=w481:errorcluster)  [unwired: 13 in]
            n121 = case shown="0, Default" w471 {
              tunnel: [1 w522] -> w501
              tunnel: w491 -> [_ w521]
              frame 0, Default {
              }
              frame 1..3 {
                n122 = Array Size(array=w521) -> (size(s)=w522:i32)
              }
            }
            n123 = call "Delay T4.vi"("milliseconds to wait"=u32 1, "error in (no error)"=w481) -> ("error out"=w493:errorcluster)  [unwired: 9 in]
            n124 = for {
              N: w501 -> [_]
              tunnel: w491 -> [w594]
              tunnel: w483 -> [w583]
              tunnel: [w592] -> w468
              tunnel: w493 -> [w591]
              tunnel: [w587] -> w502
              tunnel: w500 -> [w570]
              tunnel: w499 -> [w577]
              tunnel: w498 -> [w576]
              tunnel: w497 -> [w575]
              tunnel: w496 -> [w574]
              tunnel: w473 -> [w573]
              tunnel: [w568] -> w494
              tunnel: w477 -> [w560]
              tunnel: w490 -> [w559]
              tunnel: [w556] -> w488
              tunnel: w486 -> [w554]
              tunnel: w482 -> [w553]
              tunnel: w475 -> [w552]
              tunnel: w474 -> [w551]
              tunnel: w473 -> [w550]
              shift-right: [w544] -> _
              shift-left: dbl[] [] -> [w547]
              tunnel: w471 -> [w542]
              tunnel: w470 -> [w541]
              tunnel: [w539] -> w467
              tunnel: [w538] -> w466
              tunnel: [w537] -> w465
              tunnel: [w536] -> w463
              i -> [w540]
              stop <- w556 stop-if-true
              n125 = flat-sequence {
                tunnel: w594 -> [w648]
                tunnel: w540 -> [w647]
                tunnel: w591 -> [w649]
                tunnel: [w614] -> w588
                tunnel: [w628] -> w586
                tunnel: [w629] -> w585
                tunnel: [w630] -> w584
                tunnel: [w599] -> w582
                tunnel: [w631] -> w581
                tunnel: [w627] -> w580
                tunnel: [w626] -> w579
                tunnel: [w625] -> w578
                tunnel: w573 -> [w624]
                tunnel: [w624] -> w572
                tunnel: [w623] -> w571
                tunnel: w570 -> [w623]
                tunnel: [w622] -> w569
                tunnel: [w621] -> w566
                tunnel: [w620] -> w565
                tunnel: [w619] -> w564
                tunnel: [w609] -> w563
                tunnel: [w608] -> w562
                tunnel: [w607] -> w561
                tunnel: w560 -> [w606]
                tunnel: w559 -> [w605]
                tunnel: [w605] -> w558
                tunnel: [w604] -> w555
                tunnel: w554 -> [w604]
                tunnel: w542 -> [w602]
                tunnel: w552 -> [w601]
                tunnel: w550 -> [w600]
                tunnel: [w598] -> w549
                tunnel: w547 -> [w597]
                tunnel: [w597] -> w546
                tunnel: w542 -> [w596]
                tunnel: [w596] -> w543
                tunnel: w540 -> [w595]
                tunnel: [w747] -> w589
                tunnel: [w749] -> w587
                tunnel: [w748] -> w568
                tunnel: [w746] -> w539
                tunnel: [w745] -> w538
                tunnel: [w744] -> w537
                tunnel: w564 -> [w746]
                tunnel: w565 -> [w745]
                tunnel: w566 -> [w744]
                tunnel: w569 -> [w748]
                tunnel: w571 -> [w731]
                tunnel: w572 -> [w718]
                tunnel: w578 -> [w732]
                tunnel: w579 -> [w733]
                tunnel: w580 -> [w734]
                tunnel: w574 -> [w735]
                tunnel: w581 -> [w736]
                tunnel: w582 -> [w729]
                tunnel: w575 -> [w737]
                tunnel: w576 -> [w738]
                tunnel: w577 -> [w739]
                tunnel: w583 -> [w740]
                tunnel: w584 -> [w741]
                tunnel: w585 -> [w742]
                tunnel: w586 -> [w743]
                tunnel: w588 -> [w749]
                tunnel: w563 -> [w722]
                tunnel: w562 -> [w723]
                tunnel: w561 -> [w721]
                tunnel: w558 -> [w719]
                tunnel: [w719] -> w557
                tunnel: w555 -> [w717]
                tunnel: w553 -> [w716]
                tunnel: w551 -> [w715]
                tunnel: w549 -> [w714]
                tunnel: [w714] -> w548
                tunnel: w546 -> [w713]
                tunnel: [w713] -> w545
                tunnel: w543 -> [w712]
                tunnel: [w712] -> w536
                tunnel: w541 -> [w711]
                frame #0 {
                  w635 = FALSE ("Log (T)")
                  n126 = case shown="1..3" w602 {
                    tunnel: w649 -> [w674 w681]
                    tunnel: w648 -> [w673 _]
                    tunnel: w647 -> [w672 _]
                    tunnel: [w663 w681] -> w632
                    tunnel: [w661 w684] -> w631
                    tunnel: [w660 w679] -> w622
                    tunnel: [w655 0.0] -> w598
                    tunnel: [w659 w680] -> w614
                    tunnel: w606 -> [w657 w680]
                    tunnel: [w653 "0"] -> w599
                    tunnel: [w652 w676] -> w603
                    tunnel: w601 -> [w651 w679]
                    tunnel: w600 -> [w650 w677]
                    frame 1..3 {
                      w666 = u16 0 items=["Voltage", "Current"] ("Source Mode  (0: Voltage)")
                      n127 = Index Array(array=w673, index=w672) -> (element=w655:dbl)
                      n128 = call "Ke2400 Configure Output.vi"("Source Mode  (0: Voltage)"=w666, "error in (no error)"=w674, "Compliance  Level (0.1)"="VSA_IDD(A)", "Output Level (0)"=w655, "VISA resource name"=w657) -> ("error out"=w670:errorcluster, "VISA resource name out"=w668:refnum<visa-resource-name>)  [unwired: 5 in]
                      n129 = call "Ke2400 Enable.vi"("error in (no error)"=w670, "ON/OFF"=TRUE ("Enable Output (T: Enable)"), "VISA resource name"=w668) -> ("error out"=w671:errorcluster, "VISA resource name out"=w659:refnum<visa-resource-name>)  [unwired: 7 in]
                      n130 = Number To Fractional String(number=w655, precision (6)=i16 2) -> (F-format string=w653:string)  [unwired: 2 in]
                      n131 = call "Delay T4.vi"("milliseconds to wait"=u32 50, "error in (no error)"=w671) -> ("error out"=w658:errorcluster)  [unwired: 9 in]
                      n132 = Concatenate Strings(w650, "_Sweeping Voltage on CAP Head... ", w653) -> (w652:string)
                      n133 = call "Ke2000 Reading MilAmp.vi"("error in (no error)"=w658, "VISA resource name"=w651) -> ("error out"=w663:errorcluster, "uA"=w662:string, "VISA resource name out"=w660:refnum<visa-resource-name>)  [unwired: 7 in]
                      "CP_IDD(uA)" <- w662
                      n134 = for {
                        N: 16 -> [_]
                        tunnel: w662 -> [w675]
                        tunnel: [w675] -> w661 mode=indexing
                      }
                    }
                    frame 0, Default {
                      n135 = Concatenate Strings(w677, "_No Sweeping Voltage on CAP Head... ") -> (w676:string)
                      n136 = for {
                        N: 16 -> [_]
                        tunnel: "0" ("uA") -> [w687]
                        tunnel: [w687] -> w684 mode=indexing
                      }
                    }
                  }
                  n137 = local write "STATUS"(w603) -> ()
                  n138 = call "WS1050 16 DUT AD7747 READ.vi"("error in"=w632, "Log (T)"=w635, "DUT Mask Mode (All)"=WSVCAP_SHL_I2C_DUT_Mask_Mode_Enum."C1") -> ("error out"=w644:errorcluster, "AD7747 Values"=w646:string[][])  [unwired: 7 in]
                  n139 = for {
                    tunnel: w646 -> [w709] mode=indexing
                    tunnel: [w707] -> w615 mode=indexing
                    tunnel: w644 -> [w708]
                    tunnel: [w708] -> w643
                    n140 = Index Array(array=w709, index=1) -> (element=w707:string)
                  }
                  n141 = call "WS1050 16 DUT AD7747 READ.vi"("error in"=w643, "Log (T)"=w635, "DUT Mask Mode (All)"=WSVCAP_SHL_I2C_DUT_Mask_Mode_Enum."C2") -> ("error out"=w641:errorcluster, "AD7747 Values"=w640:string[][])  [unwired: 7 in]
                  n142 = for {
                    tunnel: w640 -> [w705] mode=indexing
                    tunnel: [w703] -> w616 mode=indexing
                    tunnel: w641 -> [w704]
                    tunnel: [w704] -> w639
                    n143 = Index Array(array=w705, index=3) -> (element=w703:string)
                  }
                  n144 = call "WS1050 16 DUT AD7747 READ.vi"("error in"=w639, "Log (T)"=w635, "DUT Mask Mode (All)"=WSVCAP_SHL_I2C_DUT_Mask_Mode_Enum."C3") -> ("error out"=w637:errorcluster, "AD7747 Values"=w636:string[][])  [unwired: 7 in]
                  n145 = for {
                    tunnel: w636 -> [w701] mode=indexing
                    tunnel: [w699] -> w633 mode=indexing
                    tunnel: w637 -> [w700]
                    tunnel: [w700] -> w634
                    n146 = Index Array(array=w701, index=5) -> (element=w699:string)
                  }
                  n147 = case shown="0" w595 {
                    tunnel: w634 -> [w691 w698]
                    tunnel: [w691 w698] -> w610
                    tunnel: w633 -> [w688 w695]
                    tunnel: w616 -> [w689 w696]
                    tunnel: w615 -> [w690 w697]
                    tunnel: [w690 w697] -> w628
                    tunnel: [w689 w696] -> w629
                    tunnel: [w688 w695] -> w630
                    tunnel: [w688 w694] -> w613
                    tunnel: [w689 w693] -> w612
                    tunnel: [w690 w692] -> w611
                    frame 0 {
                      "C3 Min_T0" <- w688
                      "C2 Min_T0" <- w689
                      "C1 Min_T0" <- w690
                    }
                    frame 1, Default {
                      n148 = local read "C3 Min_T0"() -> (w694:string[])
                      n149 = local read "C1 Min_T0"() -> (w692:string[])
                      n150 = local read "C2 Min_T0"() -> (w693:string[])
                    }
                  }
                  n151 = Build Array(w615, w616, w633) -> (w617:string[][])
                  n152 = Transpose 2D Array(2D array=w617) -> (transposed array=→"CAP_Value(pF)":string[][])
                  n153 = call "WS1050 VSA_Delta C Calculation.vi"("error in (no error)"=w610, "CAP_T"=w628, "CAP_T0"=w611) -> ("error out"=w609:errorcluster, 2:"Delta C(pF)"=w619:dbl[], 3:"Delta C(pF)"=w627:string[])  [unwired: 6 in]
                  n154 = call "WS1050 VSA_Delta C Calculation.vi"("error in (no error)"=w610, "CAP_T"=w629, "CAP_T0"=w612) -> ("error out"=w608:errorcluster, 2:"Delta C(pF)"=w620:dbl[], 3:"Delta C(pF)"=w626:string[])  [unwired: 6 in]
                  n155 = call "WS1050 VSA_Delta C Calculation.vi"("error in (no error)"=w610, "CAP_T"=w630, "CAP_T0"=w613) -> ("error out"=w607:errorcluster, 2:"Delta C(pF)"=w621:dbl[], 3:"Delta C(pF)"=w625:string[])  [unwired: 6 in]
                }
                frame #1 {
                  n156 = Get Date/Time In Seconds() -> (seconds since 1Jan1904=w728:timestamp)
                  n157 = Concatenate Strings(w718, w731) -> (w730:string)
                  n158 = Get Date/Time String(seconds (now)=w728, want seconds? (F)=TRUE) -> (date string=→"date string":string, time string=→"Previous Time":string)  [unwired: 1 in]
                  n159 = Merge Errors(w722, w723, w721) -> (w720:errorcluster)
                  n160 = call "WS1050_16 DUT VSA Save Data Ver1.0.vi"("TMN DC\\CAP Data Log File Path"=w740, "Lot#"=w739, "VSA_Delta C1(pF)"=w734, "Wafer#"=w738, "File Name"=w735, "VSA_Delta C2(pF)"=w733, "error in"=w720, "Comment"=w730, "CP Current(uA)"=w736, "VSA_IDD(A)"="NA", "HD Time(Min)"=w711, "Driver"=w718, "VSA_C1"=w743, "CP HD (V)"=w717, "VSA_C2"=w742, "SN"=w737, "VSA_C3"=w741, "Test Program"=w716, "Voltage(V)"=w729, "Stress Voltage(V)"=w715, "VSA_Delta C3(pF)"=w732) -> ("error out"=w747:errorcluster)  [unwired: 6 in]
                }
              }
              n161 = Increment(x=w540) -> (x+1=→"Running Loops":i32)
              n162 = Build Array (concatenate)(w545, w548) -> (w544:dbl[])
              n163 = call "Delay T4.vi"("milliseconds to wait"=u32 1, "error in (no error)"=w589) -> ("error out"=w592:errorcluster)  [unwired: 9 in]
              n164 = Unbundle By Name(w592) -> ("status"=w567:bool)
              n165 = Compound Arithmetic op=OR(w567, w557) -> (w556:bool)
            }
            n166 = case shown="17" w463 {
              tunnel: [w503 w509] -> w469
              tunnel: w468 -> [w503 w508]
              tunnel: w467 -> [_ w507]
              tunnel: w466 -> [_ w506]
              tunnel: w465 -> [_ w505]
              tunnel: w464 -> [_ w504]
              frame 0, Default {
              }
              frame 17 {
                n167 = case shown="1, Default" w504 {
                  tunnel: w507 -> [w513 w519]
                  tunnel: w506 -> [w512 w518]
                  tunnel: w505 -> [w511 w517]
                  tunnel: w508 -> [w510 w515]
                  tunnel: [w510 w515] -> w509
                  frame 0 {
                    n168 = Build Array(w513, w512, w511) -> (→"Delta CAP_T0(pF)":dbl[][])
                  }
                  frame 1, Default {
                    n169 = Build Array(w519, w518, w517) -> (→"Delta CAP_Tc(pF)":dbl[][])
                  }
                }
              }
            }
            n170 = Unbundle By Name(w468) -> ("status"=w489:bool)
            n171 = Or(x=w489, y=w488) -> (x .or. y?=w487:bool)
            n172 = call "Delay T4.vi"("milliseconds to wait"=u32 1, "error in (no error)"=w469) -> ("error out"=w485:errorcluster)  [unwired: 9 in]
          }
          n173 = flat-sequence {
            tunnel: w298 -> [w349]
            tunnel: [w349] -> w297
            tunnel: w295 -> [w347]
            tunnel: [w348] -> w296
            frame #0 {
              n174 = Greater Or Equal?(x=w347, y="Set HD Time \nto Complete(Min)") -> (x >= y?=w348:bool)
              "HD Time\nCompleted(Min)" <- w347
            }
          }
          n175 = Unbundle By Name(w297) -> ("status"=w300:bool)
          n176 = call "Delay T4.vi"("milliseconds to wait"=u32 50, "error in (no error)"=w297) -> ("error out"=w312:errorcluster)  [unwired: 9 in]
          n177 = Compound Arithmetic op=OR(w296, w300, w290) -> (w268:bool)
        }
        n178 = VISA Write(VISA resource name=w241, write buffer="SOUR:FUNC VOLT;VOLT:MODE FIX;RANG 100;LEV 0.0;:SENS:FUNC \"CURR\";CURR:PROT 60E-3;RANG 100E-3;:OUTP ON", error in (no error)=w232) -> (VISA resource name out=w245:refnum<visa-resource-name>, error out=w236:errorcluster)  [unwired: 1 out]
        n179 = for {
          tunnel: w235 -> [w259]
          tunnel: w237 -> [w256] mode=indexing
          shift-right: [w254] -> w231
          shift-left: w236 -> [w260]
          tunnel: [w252] -> w234
          n180 = call "E3631A_Voltage Controller updated.vi"("VISA resource name"=w259, "I_VDD(A)"=0.2, "Channel Controller"=w256, "Voltage 1"=0.0, "Voltage 2"=3.3, "error in (no error)"=w260, "Voltage 3"=-3.3) -> ("VISA resource name out"=w252:refnum<visa-resource-name>, "error out"=w255:errorcluster)  [unwired: 7 in]
          n181 = call "Delay T4.vi"("milliseconds to wait"=u32 100, "error in (no error)"=w255) -> ("error out"=w254:errorcluster)  [unwired: 9 in]
        }
        n182 = flat-sequence {
          tunnel: w231 -> [w750]
          tunnel: [w750] -> w230
          frame #0 {
            n183 = local write "STATUS"("Idle...." ("STATUS")) -> ()
            n184 = One Button Dialog(message="Test Completed") -> ()  [unwired: 1 in, 1 out]
          }
        }
      }
      frame True {
        w753 = FALSE
      }
    }
    n185 = Wait Until Next ms Multiple(millisecond multiple=u32 100) -> ()  [unwired: 1 out]
    n186 = local write "Abort"(w54) -> ()
    n187 = local write "stop"(w55) -> ()
    n188 = Unbundle By Name(w57) -> ("status"=w73:bool)
    n189 = Compound Arithmetic op=OR(w50, w73, w65) -> (w72:bool)
  }
  "Ke2000 Out" <- w24
  "PS1 Out" <- w23
  n190 = local write "Abort"(w8) -> ()
  n191 = local write "stop"(w8) -> ()
  n192 = case shown="True" w21 {
    tunnel: [w758 w760] -> w7
    tunnel: w15 -> [w758 w759]
    frame False {
    }
    frame True {
      n193 = flat-sequence {
        tunnel: w759 -> [w763]
        tunnel: [w762] -> w760
        frame #0 {
          n194 = local write "Online"(FALSE ("Online")) -> ()
          n195 = call "WSVCAP SHL Host TL Close.vi"("error in"=w763) -> ("error out"=w762:errorcluster)  [unwired: 14 in]
        }
      }
    }
  }
  "error out" <- w7
  n196 = VISA Write(VISA resource name=w16, write buffer="SOUR:FUNC VOLT;VOLT:MODE FIX;RANG 100;LEV 0.0;:SENS:FUNC \"CURR\";CURR:PROT 60E-3;RANG 100E-3;:OUTP OFF", error in (no error)=w15) -> (VISA resource name out=→"VISA resource name out":refnum<visa-resource-name>, error out=→"error out 2":errorcluster)  [unwired: 1 out]
